vi "Figuring out Vision via radio ethernet here.vi"   [LabVIEW 2016, in "Huskie Swerve.lvlib"]
uses:
  Huskie Swerve.lvlib
  <vilib>/Rock Robotics/WPI/SerialPort/WPI_SerialPort.ctl
  Refname/Sensors.ctl
  Refname/Refname to String (Sensors).vi
types:
  T1 = typedef "Huskie Swerve.lvlib/Sensors.ctl" = enum16{"Gyro", "Vision USB", "Button Pressed", "Other sensor", "Generic Sensor"}
  T2 = typedef "WPI_SerialPort.ctl" = enum16{"Onboard RS-232", "MXP TTL", "USB 1", "USB 2"}
  T3 = typedef "WPI_SerialPortRef.ctl" = cluster{"DevStatus":errorcluster, "Serial Port Name":refnum<visa-resource-name>}
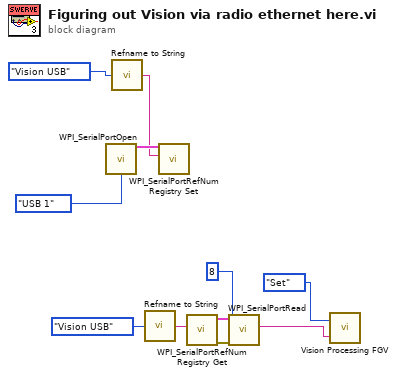
[diagram p0: block diagram]
diagram:
  n1 = call <vilib>:"WPI_SerialPortOpen.vi"("Serial Port"=WPI_SerialPort."USB 1") -> ("SerialPortRef"=w11:T3)  [unwired: 13 in, 1 out]
  n2 = call-poly "Refname to String.vi"("Enum"=Sensors."Vision USB") -> ("resulting string"=w8:string)
  n3 = call-poly "Refname to String.vi"("Enum"=Sensors."Vision USB") -> ("resulting string"=w4:string)
  n4 = call <vilib>:"WPI_SerialPortRefNum Registry Set.vi"("refnum name"=w8, "SerialPortRef"=w11) -> ()  [unwired: 8 in, 2 out]
  n5 = call <vilib>:"WPI_SerialPortRefNum Registry Get.vi"("refnum name"=w4) -> ("error out"=w7:errorcluster, "SerialPortRef"=w6:T3)  [unwired: 9 in]
  n6 = call <vilib>:"WPI_SerialPortRead.vi"("error in (no error)"=w7, "Num Bytes to Read"=u32 8, "SerialPortRef"=w6) -> ("Buffer"=w1:string)  [unwired: 6 in, 2 out]
  n7 = call "Vision Processing FGV.vi"("New Vision Processing"=w1, "Action"=enum16{"Set", "Get"}."Set") -> ()  [unwired: 1 out]
